vi "unused_new.vi"(8 "Error In":errorcluster, 10 "ref":refnum<vi>, 11 "Wire in":refnum<class "Decoration.lvclass">) -> (0 "Error Out":errorcluster, 3 "Wire Out":refnum<class "Decoration.lvclass">)   [LabVIEW 2023]
uses:
  Decoration.lvclass/Decoration.ctl
  Decoration.lvclass
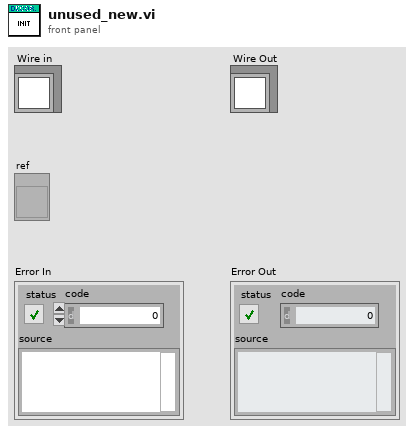
[diagram p1: front panel]
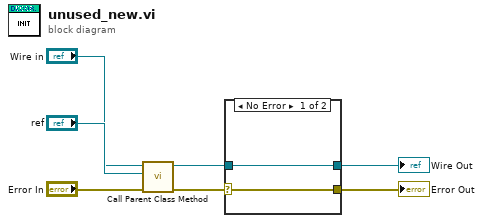
[diagram p0: block diagram]
diagram:
  n1 = call-parent "Call Parent Class Method"("Error In"="Error In", "ref"="ref", "GObject in"="Wire in") -> ("Error Out"=w4:errorcluster, "GObject out"=w1:refnum<class "Decoration.lvclass">)  [unwired: 7 in]
  n2 = case shown="No Error" w4 {
    selector: w4 -> [w9 w11]
    tunnel: [w8 w10] -> w7
    tunnel: [w9 w11] -> w6
    tunnel: w1 -> [w8 w10]
    frame No Error {
    }
    frame Error {
    }
  }
  "Wire Out" <- w7
  "Error Out" <- w6
